vi "ImagerForFlowbit5_test_cooler.vi"() -> ()   [LabVIEW 2011]
uses:
  <vilib>/Platform/TimedLoop/XDataNode/timing_clust.ctl
  <vilib>/Platform/TimedLoop/XDataNode/nitl_modes.ctl
  <vilib>/Platform/TimedLoop/XDataNode/wakeup.ctl
  <vilib>/Platform/TimedLoop/XDataNode/XDataNode.xnode
  <vilib>/Platform/TimedLoop/XDataNode/XDNodeRunTimeDep.lvlib
  <vilib>/Analysis/NI_AALBase.lvlib
panel:
  in  "开始/暂停":bool=TRUE
  in  "停止":bool
  in  "选项卡控件":T1(tab)
  out "Image 2":T2(plugin-control)
  out "循环持续时间":i64
  in  "Pra_binType":enum16{"Extract", "Resample"}(ring)
  out "数值":i32
  out "mean":dbl caption="均值" format="%0.2f"
  out "sd":dbl format="%0.2f"
  in  "Optional Rectangle":i32[](array[numeric])=[240, 240, 260, 260]
  in  "frames":i32=100
  in  "文件路径（使用对话框）":path=path "C:/Expt/test"
  in  "filename":string="test6.txt"
  out "pixel":i16
  out "mean 2":dbl caption="均值" format="%0.2f"
  out "standard deviation":dbl caption="标准差" format="%0.2f"
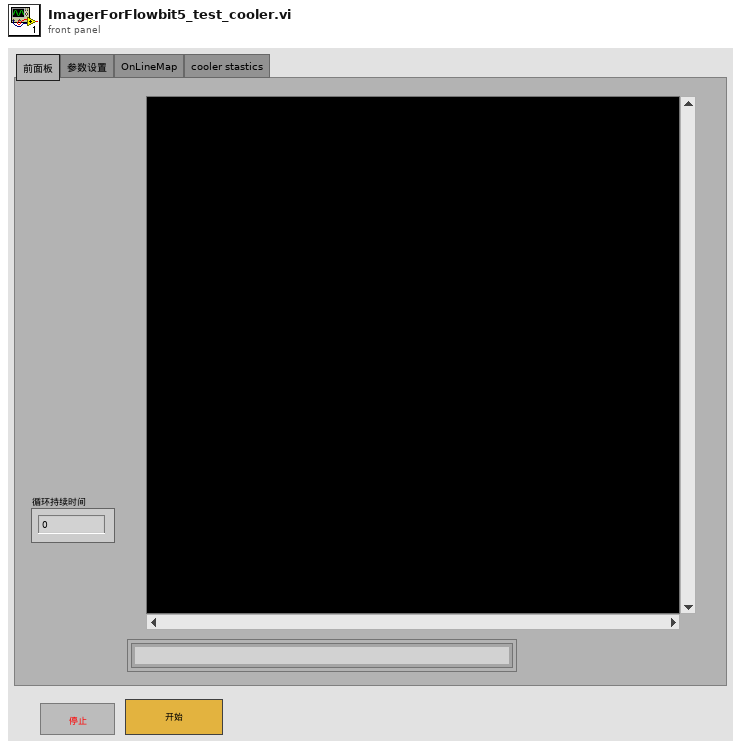
[diagram p1: front panel]
types:
  T1 = enum32{"前面板", "参数设置", "OnLineMap", "cooler stastics"}
  T2 = typedef "IMAQ Image.ctl" = refnum<image>
  T3 = enum16{"open", "replace", "create", "open or create", "replace or create", "replace or create with confirmation"}
  T4 = enum16{"Disable External Trigger", "Enable External Trigger"}
  T5 = enum32{"Auto Detect", "RoadRunner", "Raven", "R64"}
  T6 = typedef "XDNodeRunTimeDep.lvlib/timing_clust.ctl" = cluster{"Expected End [f-1]":u64, "Actual End [f-1]":u64, "Finished Late? [f-1]":bool, "Expected End [i-1]":u64, "Actual End [i-1]":u64, "Finished Late? [i-1]":bool, "Expected Start [i]":u64, "Actual Start [i]":u64, "Expected Start [f]":u64, "Actual Start [f]":u64, "Source Name":string, "Structure Name":string, "Period":i64, "Deadline":i64, "Offset":i64, "Start":i64, "Priority":i32, "Timeout":i32, "Mode":T7, "Wakeup Reason":T8, "Error":errorcluster, "Source Type":string, "Secondary Source Type":string, "Global End Time":u64, "Global Start Time":u64, "Frame Duration":u64, "Iteration Duration":u64, "Assigned CPU":i32, "I/O Scan Engine Mode":u32}
  T7 = typedef "XDNodeRunTimeDep.lvlib/nitl_modes.ctl" = enum32{"No Change", "Process missed periods, maintain original phase", "Discard missed periods, maintain original phase", "Process missed periods, ignore original phase", "Discard missed periods, ignore original phase"}
  T8 = typedef "XDNodeRunTimeDep.lvlib/wakeup.ctl" = enum32{"Normal", "Aborted", "Asynchronous wakeup", "Timing source error", "Timed loop error", "Timeout"}
  T9 = typedef "Image Type" = u32
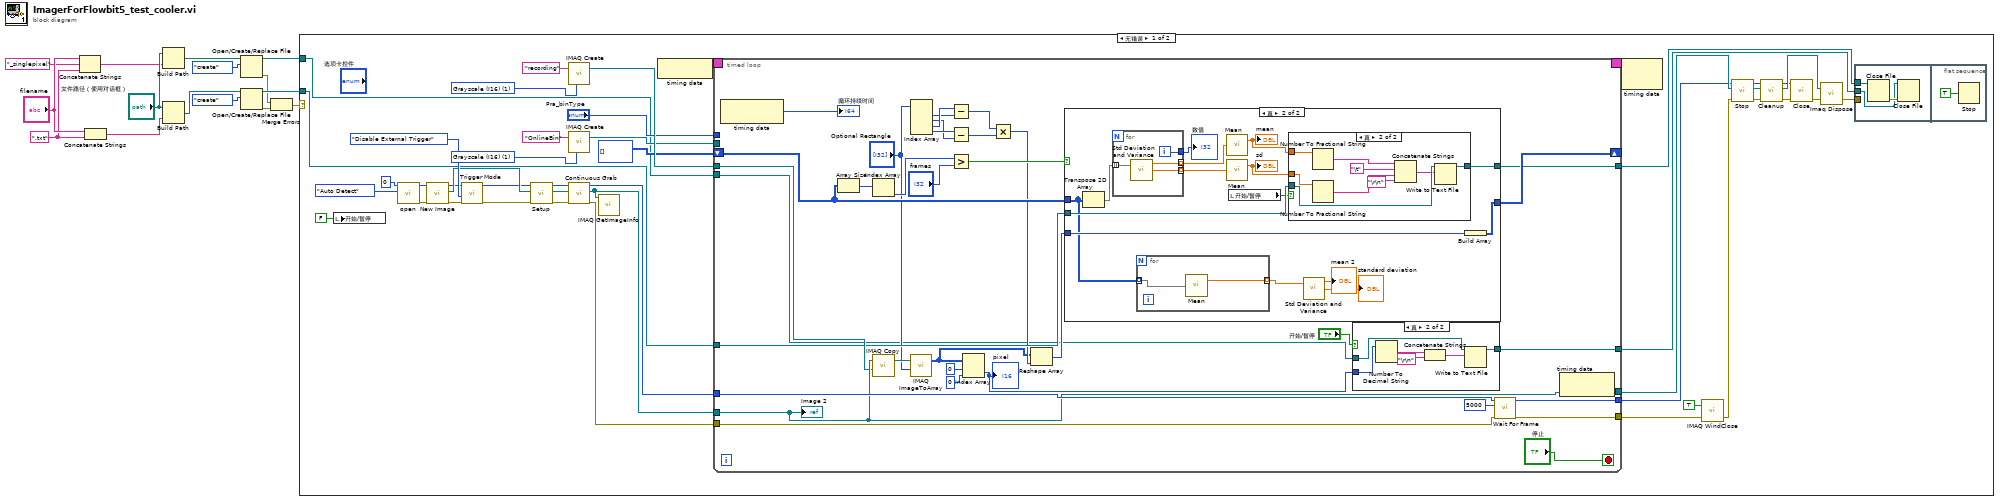
[diagram p0: block diagram]
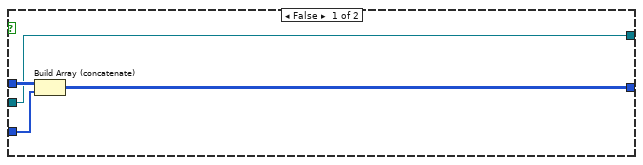
[diagram p3: hidden frame]
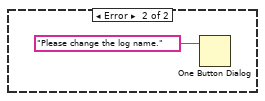
[diagram p5: hidden frame]
diagram:
  w10 = ".txt" ("字符串")
  n1 = Concatenate Strings("filename", "_singlepixel" ("字符串"), w10) -> (w7:string)
  n2 = Concatenate Strings("filename", w10) -> (w12:string)
  n3 = Build Path(base path="文件路径（使用对话框）", name or relative path=w7) -> (appended path=w5:path)
  n4 = Build Path(base path="文件路径（使用对话框）", name or relative path=w12) -> (appended path=w13:path)
  n5 = Open/Create/Replace File(file path (use dialog)=w5, operation (0:open)=T3."create" ("操作(0:open)")) -> (refnum out=w4:refnum<file>, error out=w3:errorcluster)  [unwired: 4 in, 1 out]
  n6 = Open/Create/Replace File(file path (use dialog)=w13, operation (0:open)=T3."create" ("操作(0:open)")) -> (refnum out=w14:refnum<file>, error out=w2:errorcluster)  [unwired: 4 in, 1 out]
  n7 = Merge Errors(w3, w2) -> (w1:errorcluster)
  n8 = case shown="无错误" w1 {
    tunnel: w14 -> [w20 _]
    tunnel: w4 -> [w17 _]
    frame No Error {
      w31 = T9 1 items=["Grayscale (U8)", "Grayscale (I16)", "Grayscale (SGL)", "Complex (CSG)", "RGB (U32)", "HSL (U32)", "RGB (U64)", "Grayscale (U16)"] ("Image Type")
      w33 = T9 1 items=["Grayscale (U8)", "Grayscale (I16)", "Grayscale (SGL)", "Complex (CSG)", "RGB (U32)", "HSL (U32)", "RGB (U64)", "Grayscale (U16)"] ("Image Type")
      n9 = local write "开始/暂停"(FALSE ("开始/暂停")) -> ()
      n10 = call <vilib>:"open.vi"("Board Type"=T5."Auto Detect", "Board Number"=u32 0) -> ("error out"=w47:errorcluster, "RefBrdOut"=w43:u32)  [unwired: 2 in, 5 out]
      n11 = call <vilib>:"New Image.vi"("RefBrdIn"=w43, "error in"=w47) -> ("RefBrdOut"=w42:u32, "Image"=w55:T2, "error out"=w48:errorcluster)  [unwired: 6 in]
      n12 = call <vilib>:"Trigger Mode.vi"("RefBrdIn"=w42, "Trigger Mode"=T4."Disable External Trigger", "error in (no error)"=w48) -> ("RefBrdOut"=w41:u32, "error out"=w49:errorcluster)  [unwired: 6 in]
      n13 = call <vilib>:"Setup.vi"("error in"=w49, "Image In"=w55, "RefBrdIn"=w41) -> ("error out"=w44:errorcluster, "Image"=w45:T2, "RefBrdOut"=w40:u32)  [unwired: 6 in]
      n14 = call "IMAQ Create"("Image Name"="recording", "Image Type"=w33) -> ("New Image"=w35:T2)  [unwired: 3 in, 1 out]
      n15 = call "IMAQ Create"("Image Name"="OnlineBin", "Image Type"=w31) -> ("New Image"=w30:T2)  [unwired: 3 in, 1 out]
      n16 = call <vilib>:"Continuous Grab.vi"("error in (no error)"=w44, "Image In"=w45, "RefBrdIn"=w40) -> ("error out"=w23:errorcluster, "Image"=w28:T2, "RefBrdOut"=w24:u32)  [unwired: 6 in]
      n17 = call "IMAQ GetImageInfo"("Image"=w28) -> ()  [unwired: 3 in, 8 out]
      n18 = node-c288() -> (w59:T6)
      n19 = timed-loop {
        tunnel: [w91] -> w54
        tunnel: [w97] -> w27
        tunnel: w28 -> [w91]
        tunnel: w23 -> [w96]
        tunnel: w24 -> [w95]
        tunnel: [w94] -> w39
        timing: w59 -> [_]
        timing-out: [_] -> w58
        tunnel: w35 -> [w90]
        tunnel: w30 -> [_]
        tunnel: "Pra_binType" -> [_]
        shift-right: [w87] -> _
        shift-left: i16[][] [] -> [w88]
        tunnel: w20 -> [w86]
        tunnel: [w85] -> w19
        tunnel: w17 -> [w65]
        tunnel: [w64] -> w16
        stop <- "停止" stop-if-true
        n20 = node-c288() -> (→"循环持续时间":i64)  [unwired: 1 in]
        n21 = Array Size(array=w88) -> (size(s)=w82:i32[])
        n22 = Index Array(array=w82) -> (element=w81:i32)  [unwired: 1 in]
        n23 = call "IMAQ Copy"("Image Dst"=w90, "Image Src"=w91) -> ("Image Dst Out"=w84:T2)  [unwired: 4 in, 1 out]
        n24 = call "IMAQ ImageToArray"("Optional Rectangle"="Optional Rectangle", "Image"=w84) -> ("Image Pixels (I16)"=w70:i16[][])  [unwired: 2 in, 4 out]
        n25 = Index Array(array="Optional Rectangle") -> (element #1=w76:i32, element #2=w74:i32, element #3=w77:i32, element #4=w75:i32)  [unwired: 4 in]
        n26 = Subtract(x=w77, y=w76) -> (x-y=w72:i32)
        n27 = Subtract(x=w75, y=w74) -> (x-y=w73:i32)
        n28 = Greater?(x=w81, y="frames") -> (0:w79:bool)
        n29 = Index Array(array=w70, index (row)=0 ("禁用的索引 (行)"), index (col)=0 ("禁用的索引 (列)")) -> (element=w66:i16)
        "pixel" <- w66
        n30 = Multiply(x=w72, y=w73) -> (x*y=w71:i32)
        n31 = Reshape Array(w70, w71) -> (w83:i16[])
        n32 = case shown="真" w79 {
          tunnel: w83 -> [w108 w119]
          tunnel: [w106 w118] -> w87
          tunnel: w88 -> [w107 w112]
          tunnel: w86 -> [w105 w117]
          tunnel: [w105 w114] -> w85
          frame False {
            n33 = Build Array (concatenate)(w107, w108) -> (w106:i16[][])
          }
          frame True {
            n34 = Transpose 2D Array(2D array=w112) -> (transposed array=w123:i16[][])
            n35 = for {
              tunnel: w123 -> [w138] mode=indexing
              tunnel: [w139] -> w122
              tunnel: [w137] -> w121 mode=indexing
              tunnel: [w136] -> w120 mode=indexing
              i -> [w139]
              n36 = call <vilib>:"Std Deviation and Variance.vi"("X"=w138) -> ("mean"=w137:dbl, "standard deviation"=w136:dbl)  [unwired: 1 in, 1 out]
            }
            "数值" <- w122
            n37 = for {
              tunnel: w112 -> [w125] mode=indexing
              tunnel: [w124] -> w111 mode=indexing
              n38 = call <vilib>:"Mean.vi"("X"=w125) -> ("mean"=w124:dbl)  [unwired: 1 out]
            }
            n39 = call <vilib>:"Mean.vi"("X"=w121) -> ("mean"=w116:dbl)  [unwired: 1 out]
            "mean" <- w116
            n40 = call <vilib>:"Mean.vi"("X"=w120) -> ("mean"=w115:dbl)  [unwired: 1 out]
            "sd" <- w115
            n41 = local read "开始/暂停"() -> (w113:bool)
            n42 = case shown="真" w113 {
              tunnel: w117 -> [w126 w135]
              tunnel: w116 -> [_ w132]
              tunnel: w115 -> [_ w130]
              tunnel: [w126 w127] -> w114
              frame False {
              }
              frame True {
                n43 = Number To Fractional String(number=w132) -> (F-format string=w131:string)  [unwired: 3 in]
                n44 = Number To Fractional String(number=w130) -> (F-format string=w129:string)  [unwired: 3 in]
                n45 = Concatenate Strings(w131, "\t", w129, "\r\n") -> (w128:string)
                n46 = Write to Text File(file (use dialog)=w135, text=w128) -> (refnum out=w127:refnum<file>)  [unwired: 2 in, 2 out]
              }
            }
            n47 = call <vilib>:"Std Deviation and Variance.vi"("X"=w111) -> ("mean"=→"mean 2":dbl, "standard deviation"=→"standard deviation":dbl)  [unwired: 1 in, 1 out]
            n48 = Build Array(w119) -> (w118:i16[][])
          }
        }
        n49 = case shown="真" "开始/暂停" {
          tunnel: w66 -> [_ w103]
          tunnel: w65 -> [w98 w101]
          tunnel: [w98 w100] -> w64
          frame False {
          }
          frame True {
            n50 = Number To Decimal String(number=w103) -> (decimal integer string=w102:string)  [unwired: 1 in]
            n51 = Concatenate Strings(w102, "\r\n") -> (w99:string)
            n52 = Write to Text File(file (use dialog)=w101, text=w99) -> (refnum out=w100:refnum<file>)  [unwired: 2 in, 2 out]
          }
        }
        n53 = call <vilib>:"Wait For Frame.vi"("error in (no error)"=w96, "Timeout (mS)"=u32 5000, "RefBrdIn"=w95) -> ("error out"=w97:errorcluster, "RefBrdOut"=w94:u32)  [unwired: 7 in]
        n54 = node-c288() -> ()  [unwired: 1 in, 1 out]
        "Image 2" <- w91
      }
      n55 = node-c288(w58) -> ()  [unwired: 1 out]
      n56 = call "IMAQ WindClose"("Close All Windows (False)"=TRUE, "error in (no error)"=w27) -> ("error out"=w26:errorcluster)  [unwired: 4 in]
      n57 = call <vilib>:"Stop.vi"("error in (no error)"=w26, "Image In"=w54, "RefBrdIn"=w39) -> ("error out"=w50:errorcluster, "Image"=w53:T2, "RefBrdOut"=w38:u32)  [unwired: 6 in]
      n58 = call <vilib>:"Cleanup.vi"("error in (no error)"=w50, "Image In"=w53, "RefBrdIn"=w38) -> ("error out"=w51:errorcluster, "Image"=w52:T2, "RefBrdOut"=w37:u32)  [unwired: 6 in]
      n59 = call <vilib>:"Close.vi"("error in (no error)"=w51, "RefBrdIn"=w37) -> ("error out"=w36:errorcluster)  [unwired: 8 in, 1 out]
      n60 = call "Imaq Dispose"("Image"=w52, "error in (no error)"=w36) -> ("error out"=w22:errorcluster)  [unwired: 4 in]
      n61 = flat-sequence {
        tunnel: w22 -> [_]
        tunnel: w19 -> [w62]
        tunnel: w16 -> [w60]
        frame #0 {
          n62 = Close File(refnum=w62) -> (error out=w61:errorcluster)  [unwired: 1 in, 1 out]
          n63 = Close File(refnum=w60, error in=w61) -> ()  [unwired: 2 out]
        }
        frame #1 {
          n64 = Stop(stop? (T)=TRUE ("停止？(T)")) -> ()
        }
      }
    }
    frame Error {
      n65 = One Button Dialog(message="Please change the log name." ("消息")) -> ()  [unwired: 1 in, 1 out]
    }
  }
